vi "NIDAQ-AO-PS_Core.vi"(8 "error in":errorcluster, 10 "ctrl queue in":refnum<queue>) -> (0 "error out":errorcluster, 2 "ctrl queue out":refnum<queue>)   [LabVIEW 2014, in "NIDAQ_AO_PowerSupply.lvlib"]
uses:
  <instrlib>/NIDAQmxAOPowerSupply/NIDAQ_AO_PowerSupply.lvlib
  <instrlib>/GenericDCPowerSupply/Public/GenericDCPS-State.ctl
  <instrlib>/GenericDCPowerSupply/Public/Data/HVCh-Configs.ctl
  <vilib>/Utility/error.llb/Error Cluster From Error Code.vi
  <vilib>/DAQmx/write.llb/DAQmx Write.vi
  <vilib>/DAQmx/write.llb/DAQmx Write (Analog 1D DBL NChan 1Samp).vi
  <vilib>/ErrorRing/Error Ring.xnode
  <userlib>/Utility/ErrorLog_lib.lvlib
  <instrlib>/GenericDCPowerSupply/GenericDCPowerSupply.lvlib
panel:
  out "Power Supply Monitoring":cluster{"Gauge":dbl, "Clamped":bool}[][](array[cluster]) {"Gauge" scale=0.0..5000.0 scale format="%#_6p"}
  in  "Configs":T2={"Enable"=FALSE, "ZeroShutdown"=FALSE, "Initialized"=FALSE, "Configs"=[{"MaxVolt"=5.0, "MinVolt"=0.0, "SetPoint"=0.0, "Readout"=0.0, "Enable"=TRUE, "Channel"=0, "Clamped"=FALSE}, {"MaxVolt"=5.0, "MinVolt"=0.0, "SetPoint"=0.0, "Readout"=0.0, "Enable"=TRUE, "Channel"=1, "Clamped"=FALSE}, {"MaxVolt"=5.0, "MinVolt"=0.0, "SetPoint"=0.0, "Readout"=0.0, "Enable"=TRUE, "Channel"=2, "Clamped"=FALSE}, {"MaxVolt"=5.0, "MinVolt"=0.0, "SetPoint"=0.0, "Readout"=0.0, "Enable"=TRUE, "Channel"=3, "Clamped"=FALSE}, {"MaxVolt"=5.0, "MinVolt"=0.0, "SetPoint"=0.0, "Readout"=0.0, "Enable"=TRUE, "Channel"=4, "Clamped"=FALSE}, {"MaxVolt"=5.0, "MinVolt"=0.0, "SetPoint"=0.0, "Readout"=0.0, "Enable"=TRUE, "Channel"=5, "Clamped"=FALSE}, {"MaxVolt"=5.0, "MinVolt"=0.0, "SetPoint"=0.0, "Readout"=0.0, "Enable"=TRUE, "Channel"=6, "Clamped"=FALSE}, {"MaxVolt"=5.0, "MinVolt"=0.0, "SetPoint"=0.0, "Readout"=0.0, "Enable"=TRUE, "Channel"=7, "Clamped"=FALSE}, {"MaxVolt"=5.0, "MinVolt"=0.0, "SetPoint"=0.0, "Readout"=0.0, "Enable"=TRUE, "Channel"=8, "Clamped"=FALSE}, {"MaxVolt"=5.0, "MinVolt"=0.0, "SetPoint"=0.0, "Readout"=0.0, "Enable"=TRUE, "Channel"=9, "Clamped"=FALSE}, {"MaxVolt"=5.0, "MinVolt"=0.0, "SetPoint"=0.0, "Readout"=0.0, "Enable"=TRUE, "Channel"=10, "Clamped"=FALSE}, {"MaxVolt"=5.0, "MinVolt"=0.0, "SetPoint"=0.0, "Readout"=0.0, "Enable"=TRUE, "Channel"=11, "Clamped"=FALSE}, {"MaxVolt"=5.0, "MinVolt"=0.0, "SetPoint"=0.0, "Readout"=0.0, "Enable"=TRUE, "Channel"=12, "Clamped"=FALSE}, {"MaxVolt"=5.0, "MinVolt"=0.0, "SetPoint"=0.0, "Readout"=0.0, "Enable"=TRUE, "Channel"=13, "Clamped"=FALSE}, {"MaxVolt"=5.0, "MinVolt"=0.0, "SetPoint"=0.0, "Readout"=0.0, "Enable"=TRUE, "Channel"=14, "Clamped"=FALSE}, {"MaxVolt"=5.0, "MinVolt"=0.0, "SetPoint"=0.0, "Readout"=0.0, "Enable"=TRUE, "Channel"=15, "Clamped"=FALSE}], "AO Task Name"="", "# Channels"=16, "Actual Ctrl Voltages"=[]}
  in  "Quit":bool
  in  "SetAll":bool
  # "Copyright (C) 2015 MassThink.\nCopyright (C) 2015 University of Illinois at Chicago\nLicensed under LGPL v3.\n\nProvided AS IS, use at your own risk.\n\nHardware overvoltage protection \nmust be used."
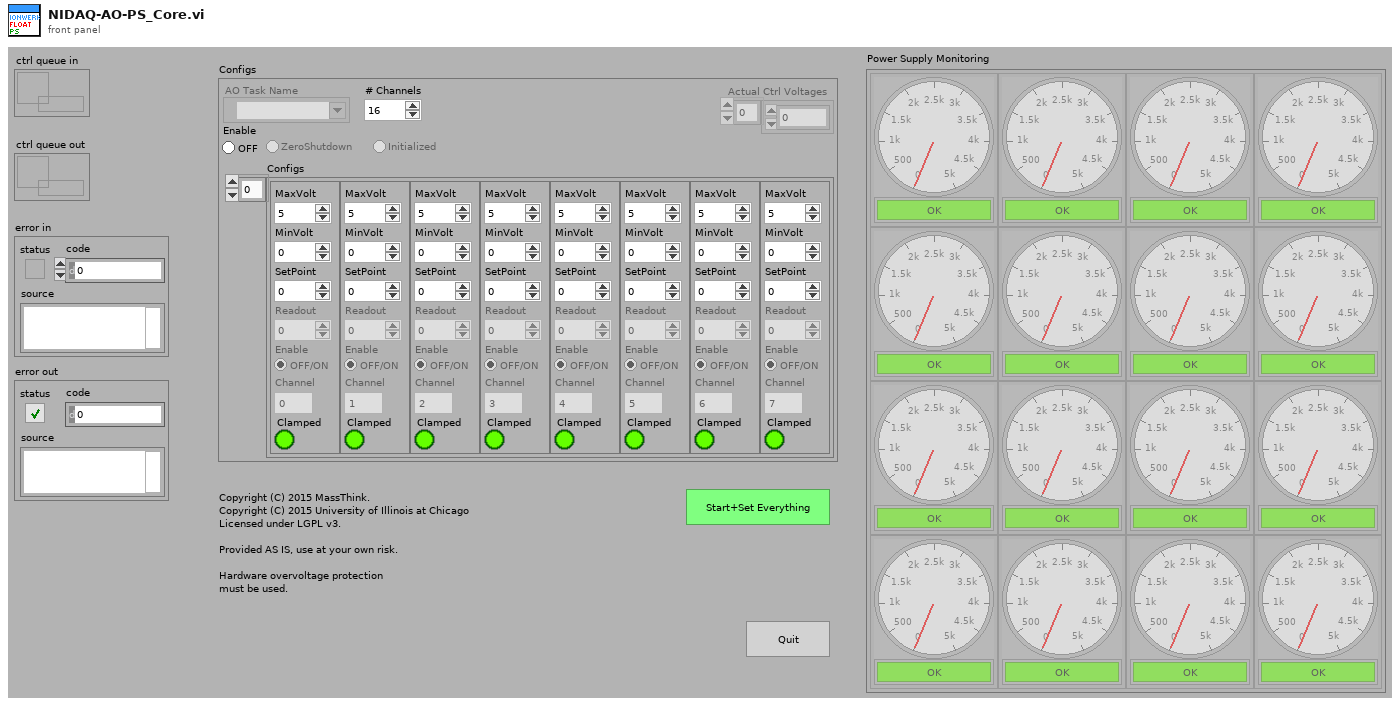
[diagram p1: front panel]
types:
  T1 = typedef "GenericDCPowerSupply.lvlib/HVCh-Configs.ctl" = cluster{"MaxVolt":dbl, "MinVolt":dbl, "SetPoint":dbl, "Readout":dbl, "Enable":bool, "Channel":i32, "Clamped":bool}
  T2 = cluster{"Enable":bool, "ZeroShutdown":bool, "Initialized":bool, "Configs":T1[], "AO Task Name":refnum<k21>, "# Channels":i32, "Actual Ctrl Voltages":dbl[]}
  T3 = enum8{"Enabled", "Disabled", "Disabled and Grayed Out"}
  T4 = cluster{"Slope(Output)":dbl, "Offset(Output)":dbl, "Slope(Input)":dbl, "Offset(Input)":dbl}[][]
  T5 = cluster{"Slope(Output)":dbl, "Offset(Output)":dbl, "Slope(Input)":dbl, "Offset(Input)":dbl}[]
  T6 = typedef "GenericDCPowerSupply.lvlib/GenericDCPS-State.ctl" = cluster{"State":enum16{"Enurmerate", "Open", "WriteVoltage", "ReadVoltage", "WriteAllChs", "ReadAllChs", "OnOff", "SetMinMax", "Close", "Quit", "=========", "GetStatus"}, "Para.":variant}
  T7 = enum16{"Enurmerate", "Open", "WriteVoltage", "ReadVoltage", "WriteAllChs", "ReadAllChs", "OnOff", "SetMinMax", "Close", "Quit", "=========", "GetStatus"}
  T8 = cluster{"Slope(Output)":dbl, "Offset(Output)":dbl, "Slope(Input)":dbl, "Offset(Input)":dbl}
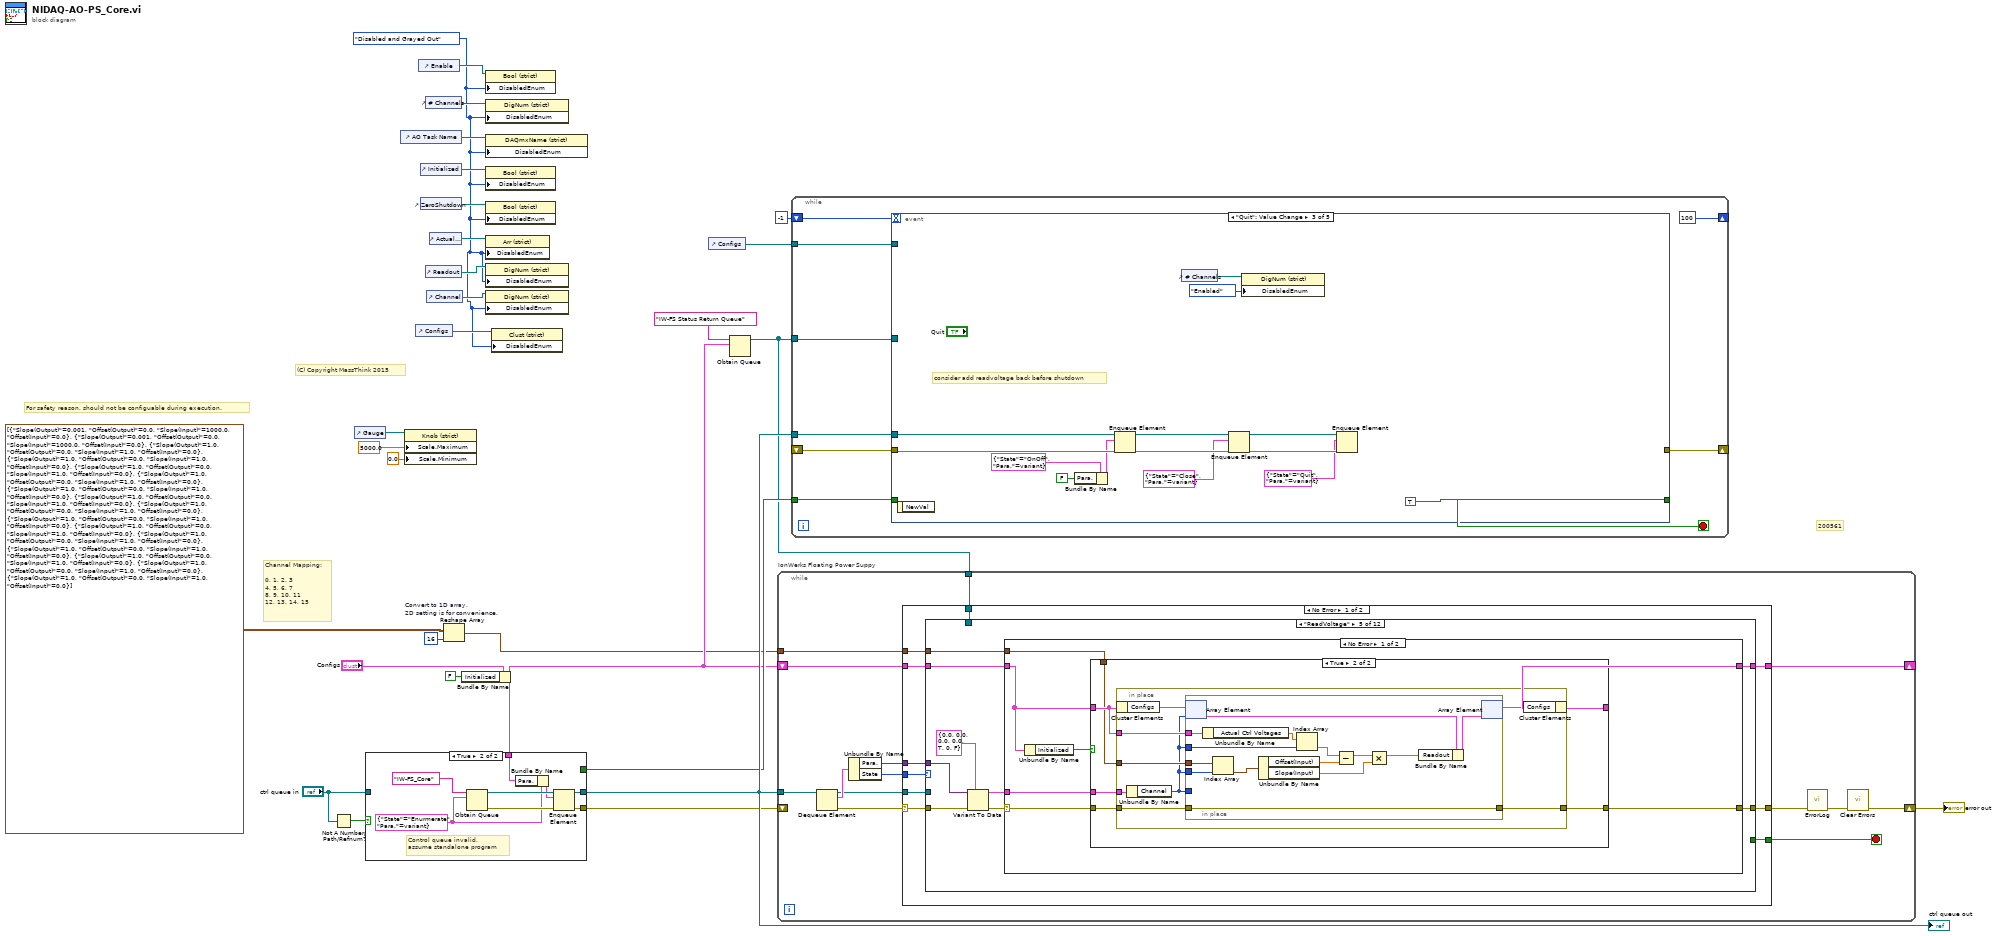
[diagram p0: block diagram]
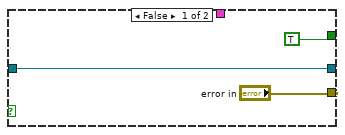
[diagram p2: hidden frame]
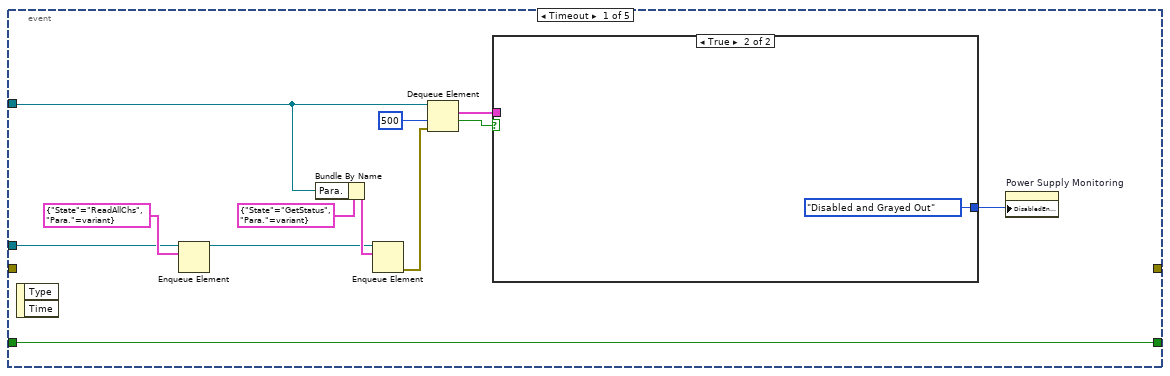
[diagram p3: hidden frame]
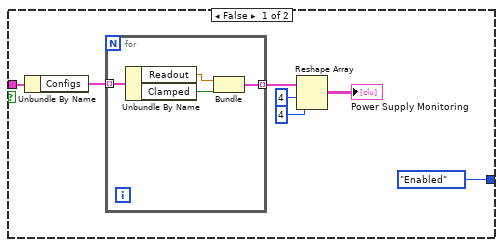
[diagram p4: hidden frame]
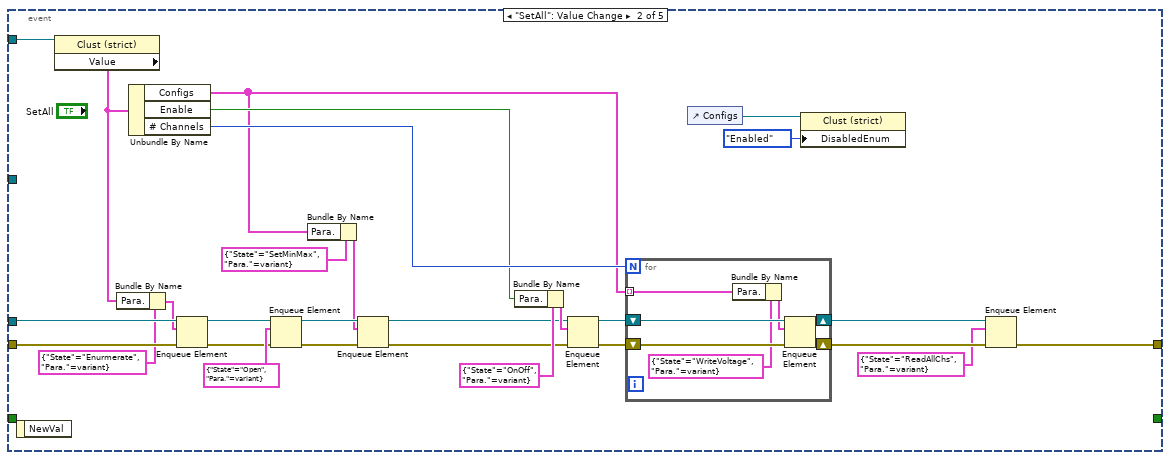
[diagram p5: hidden frame]
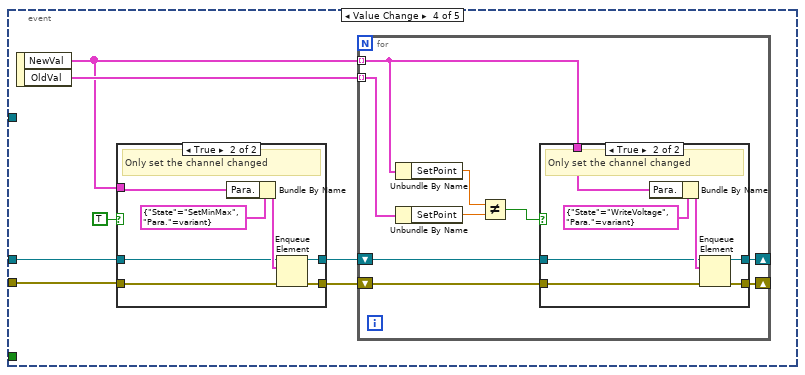
[diagram p6: hidden frame]
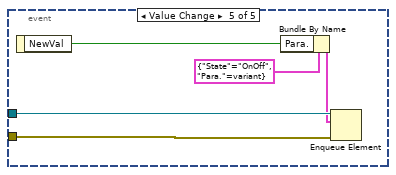
[diagram p9: hidden frame]
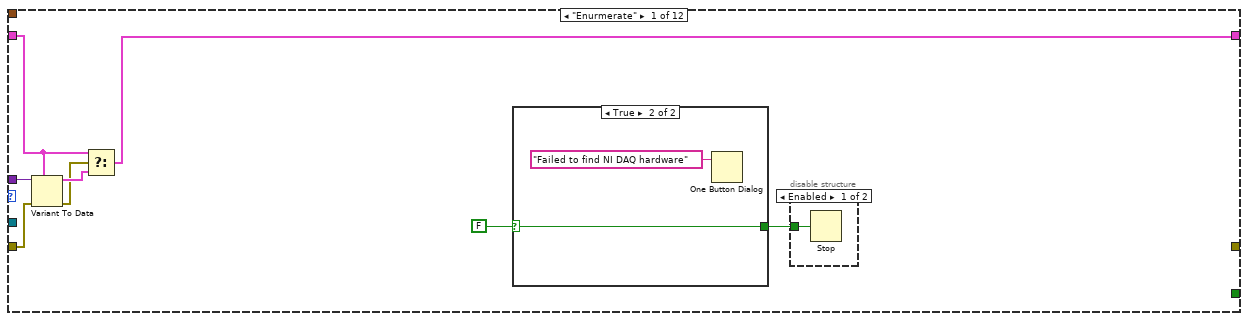
[diagram p10: hidden frame]
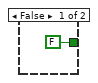
[diagram p12: hidden frame]
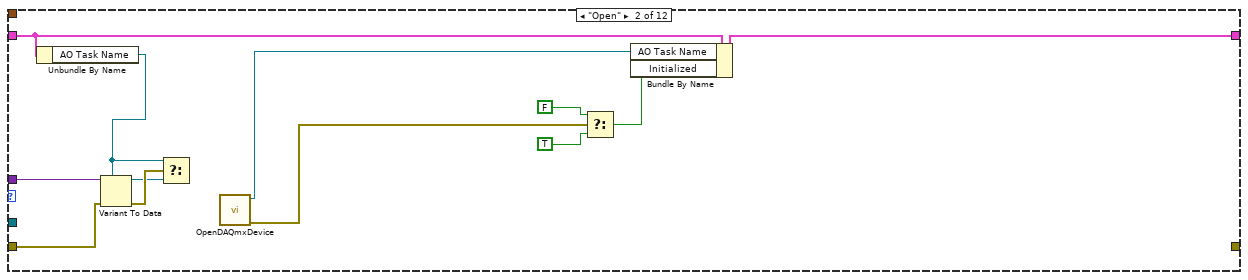
[diagram p13: hidden frame]
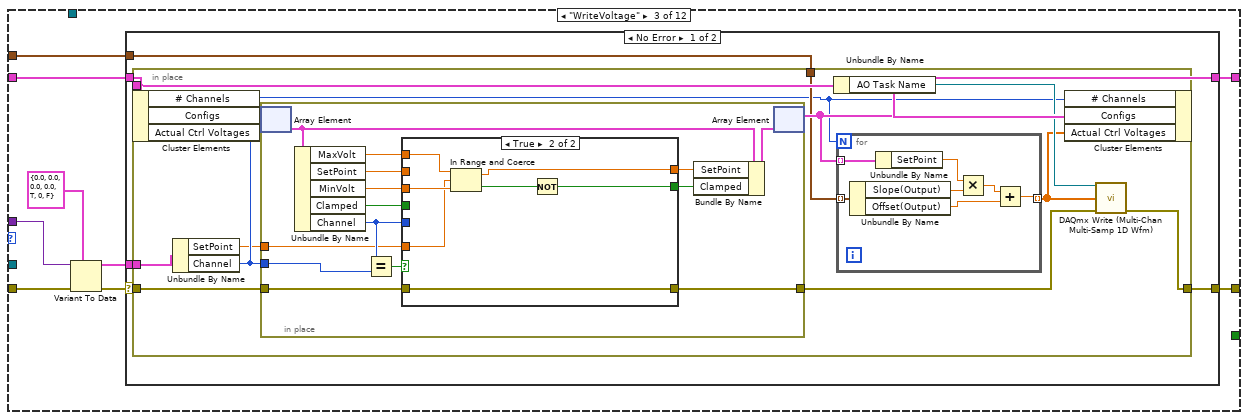
[diagram p14: hidden frame]
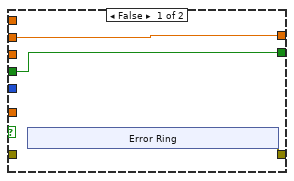
[diagram p15: hidden frame]
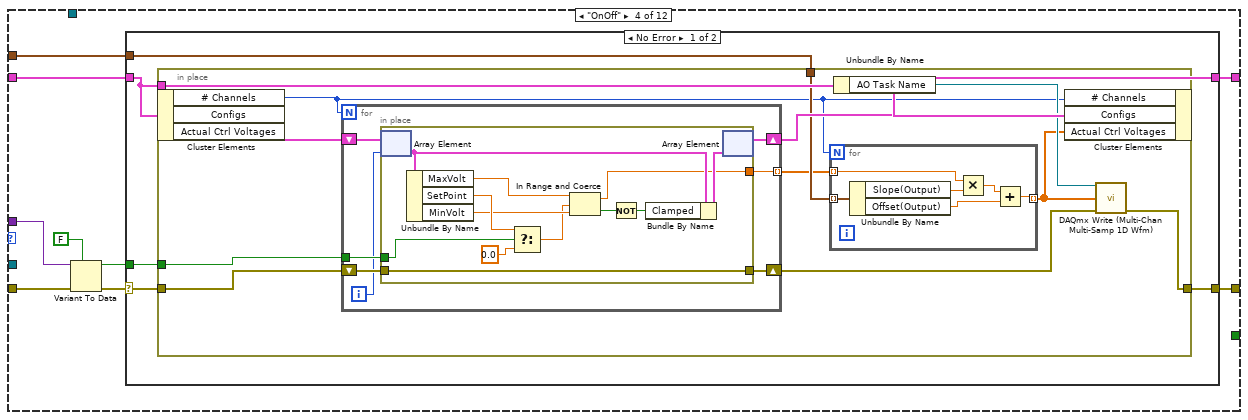
[diagram p17: hidden frame]
diagram:
  w1 = T3."Disabled and Grayed Out" ("Disabled")
  # "200561"
  # "Channel Mapping:\n\n0, 1, 2, 3\n4, 5, 6, 7\n8, 9, 10, 11\n12, 13, 14, 15"
  # "For safety reason, should not be configuable during execution."
  # "(C) Copyright MassThink 2015"
  n1 = Not A Number/Path/Refnum?(number/path/refnum="ctrl queue in") -> (NaN/Path/Refnum?=w28:bool)
  n2 = control-ref of="Gauge"() -> (w20:refnum<vi>)
  n3 = control-ref of="AO Task Name"() -> (w6:refnum<vi>)
  n4 = property class="Knob (strict)"(reference=w20, "Scale.Maximum"=5000.0 ("Scale.Range:Maximum"), "Scale.Minimum"=0.0 ("Scale.Range:Minimum")) -> ()  [unwired: 1 in, 2 out]
  n5 = control-ref of="Configs"() -> (w2:refnum<vi>)
  n6 = control-ref of="Enable"() -> (w5:refnum<vi>)
  n7 = control-ref of="Initialized"() -> (w7:refnum<vi>)
  n8 = control-ref of="ZeroShutdown"() -> (w8:refnum<vi>)
  n9 = control-ref of="# Channels"() -> (w10:refnum<vi>)
  n10 = control-ref of="Readout"() -> (w3:refnum<vi>)
  n11 = control-ref of="Channel"() -> (w4:refnum<vi>)
  n12 = control-ref of="Actual Ctrl Voltages"() -> (w9:refnum<vi>)
  n13 = Reshape Array "Convert to 1D array,\n2D setting is for convenience."(T4 [[{"Slope(Output)"=0.001, "Offset(Output)"=0.0, "Slope(Input)"=1000.0, "Offset(Input)"=0.0}, {"Slope(Output)"=0.001, "Offset(Output)"=0.0, "Slope(Input)"=1000.0, "Offset(Input)"=0.0}, {"Slope(Output)"=1.0, "Offset(Output)"=0.0, "Slope(Input)"=1.0, "Offset(Input)"=0.0}, {"Slope(Output)"=1.0, "Offset(Output)"=0.0, "Slope(Input)"=1.0, "Offset(Input)"=0.0}], [{"Slope(Output)"=1.0, "Offset(Output)"=0.0, "Slope(Input)"=1.0, "Offset(Input)"=0.0}, {"Slope(Output)"=1.0, "Offset(Output)"=0.0, "Slope(Input)"=1.0, "Offset(Input)"=0.0}, {"Slope(Output)"=1.0, "Offset(Output)"=0.0, "Slope(Input)"=1.0, "Offset(Input)"=0.0}, {"Slope(Output)"=1.0, "Offset(Output)"=0.0, "Slope(Input)"=1.0, "Offset(Input)"=0.0}], [{"Slope(Output)"=1.0, "Offset(Output)"=0.0, "Slope(Input)"=1.0, "Offset(Input)"=0.0}, {"Slope(Output)"=1.0, "Offset(Output)"=0.0, "Slope(Input)"=1.0, "Offset(Input)"=0.0}, {"Slope(Output)"=1.0, "Offset(Output)"=0.0, "Slope(Input)"=1.0, "Offset(Input)"=0.0}, {"Slope(Output)"=1.0, "Offset(Output)"=0.0, "Slope(Input)"=1.0, "Offset(Input)"=0.0}], [{"Slope(Output)"=1.0, "Offset(Output)"=0.0, "Slope(Input)"=1.0, "Offset(Input)"=0.0}, {"Slope(Output)"=1.0, "Offset(Output)"=0.0, "Slope(Input)"=1.0, "Offset(Input)"=0.0}, {"Slope(Output)"=1.0, "Offset(Output)"=0.0, "Slope(Input)"=1.0, "Offset(Input)"=0.0}, {"Slope(Output)"=1.0, "Offset(Output)"=0.0, "Slope(Input)"=1.0, "Offset(Input)"=0.0}]] ("output array"), 16 ("dimension size")) -> (w11:T5)
  n14 = Bundle By Name(cluster="Configs", "Initialized"=FALSE) -> (w17:T2)
  n15 = case shown="True" w28 {
    tunnel: [w32 w37] -> w27
    tunnel: ["error in" w39] -> w26
    tunnel: "ctrl queue in" -> [w32 _]
    tunnel: w17 -> [_ w34]
    tunnel: [TRUE _] -> w25
    frame False {
    }
    frame True {
      w33 = T6 {"State"=enum."Enurmerate", "Para."=variant}
      # "Control queue invalid, \nassume standalone program"
      n16 = Obtain Queue(name (unnamed)="IW-FS_Core", element data type=w33) -> (queue out=w38:refnum<queue>, error out=w39:errorcluster)  [unwired: 3 in, 1 out]
      n17 = Bundle By Name(cluster=w33, "Para."=w34) -> (w35:T6)
      n18 = Enqueue Element(queue=w38, element=w35) -> (queue out=w37:refnum<queue>)  [unwired: 2 in, 2 out]
    }
  }
  "ctrl queue out" <- w27
  n19 = property class="Bool (strict)"(reference=w5, "DisabledEnum"=w1) -> ()  [unwired: 1 in, 2 out]
  n20 = property class="DigNum (strict)"(reference=w10, "DisabledEnum"=w1) -> ()  [unwired: 1 in, 2 out]
  n21 = property class="DAQmxName (strict)"(reference=w6, "DisabledEnum"=w1) -> ()  [unwired: 1 in, 2 out]
  n22 = property class="Bool (strict)"(reference=w7, "DisabledEnum"=w1) -> ()  [unwired: 1 in, 2 out]
  n23 = property class="Bool (strict)"(reference=w8, "DisabledEnum"=w1) -> ()  [unwired: 1 in, 2 out]
  n24 = property class="Arr (strict)"(reference=w9, "DisabledEnum"=w1) -> ()  [unwired: 1 in, 2 out]
  n25 = property class="DigNum (strict)"(reference=w3, "DisabledEnum"=w1) -> ()  [unwired: 1 in, 2 out]
  n26 = property class="DigNum (strict)"(reference=w4, "DisabledEnum"=w1) -> ()  [unwired: 1 in, 2 out]
  n27 = property class="Clust (strict)"(reference=w2, "DisabledEnum"=w1) -> ()  [unwired: 1 in, 2 out]
  n28 = control-ref of="Configs"() -> (w15:refnum<vi>)
  n29 = Obtain Queue(name (unnamed)="IW-FS Status Return Queue", element data type=w17) -> (queue out=w18:refnum<queue>)  [unwired: 3 in, 2 out]
  n30 = while "IonWerks Floating Power Suppy" {
    tunnel: w27 -> [w53]
    shift-right: [w44] -> w29
    shift-left: w26 -> [_]
    shift-right: [w45] -> _
    shift-left: w17 -> [w46]
    tunnel: w18 -> [w41]
    tunnel: w11 -> [w40]
    stop <- w47 stop-if-true
    n31 = Dequeue Element(queue=w53) -> (queue out=w49:refnum<queue>, element=w52:T6, error out=w48:errorcluster)  [unwired: 2 in, 1 out]
    n32 = Unbundle By Name(w52) -> ("Para."=w50:variant, "State"=w51:T7)
    n33 = case shown="No Error" w48 {
      selector: w48 -> [w57 w359]
      tunnel: w51 -> [w63 _]
      tunnel: w50 -> [w62 _]
      tunnel: w49 -> [w61 _]
      tunnel: [w60 w359] -> w42
      tunnel: [w56 TRUE] -> w47
      tunnel: w46 -> [w59 w360]
      tunnel: [w58 w360] -> w45
      tunnel: w41 -> [w55 _]
      tunnel: w40 -> [w54 _]
      frame No Error {
        n34 = case shown="\"ReadVoltage\"" w63 {
          tunnel: w62 -> [w71 w87 w95 w162 w215 _ _ w286 _ _ _ w352]
          tunnel: w61 -> [_ _ _ _ _ _ _ _ _ _ _ _]
          tunnel: w57 -> [w70 w85 w94 w161 w214 w258 w263 w285 w329 w348 w350 w354]
          tunnel: [_ _ w89 w156 w210 w258 w262 w283 w328 w348 w350 w353] -> w60
          tunnel: w59 -> [w68 w84 w91 w158 w209 w257 w267 w280 w330 w347 w349 w356]
          tunnel: [w66 w86 w90 w157 w211 w257 w265 w279 w326 w347 w349 w356] -> w58
          tunnel: [_ _ _ _ _ _ _ _ _ TRUE _ _] -> w56
          tunnel: w55 -> [_ _ _ _ _ _ _ _ _ _ _ w351]
          tunnel: w54 -> [_ _ w88 w155 w208 _ w259 _ _ _ _ _]
          frame "Enurmerate" {
            n35 = Variant To Data(error in=w70, type=w68, Variant=w71) -> (data=w69:T2, error out=w67:errorcluster)
            n36 = Select(t=w68, s=w67, f=w69) -> (s? t:f=w66:T2)
            n37 = case shown="True" FALSE ("status") {
              selector: FALSE ("status") -> [_ w74]
              tunnel: [FALSE w74] -> w65
              frame False {
              }
              frame True {
                n38 = One Button Dialog(message="Failed to find NI DAQ hardware") -> ()  [unwired: 1 in, 1 out]
              }
            }
            n39 = disable-structure shown="Enabled" {
              disable-tunnel: w65 -> [w72 _]
              frame Enabled {
                n40 = Stop(stop? (T)=w72) -> ()
              }
              frame Disabled {
              }
            }
          }
          frame "Open" {
            n41 = Unbundle By Name(w84) -> ("AO Task Name"=w82:refnum<k21>)
            n42 = Variant To Data(error in=w85, type=w82, Variant=w87) -> (data=w81:refnum<k21>, error out=w83:errorcluster)
            n43 = Select(t=w82, s=w83, f=w81) -> ()  [unwired: 1 out]
            n44 = call <instrlib>:"OpenDAQmxDevice.vi"() -> ("error out"=w76:errorcluster, "task out"=w77:refnum<k21>)  [unwired: 9 in, 1 out]
            n45 = Select(t=FALSE ("x < y?"), s=w76, f=TRUE ("x < y?")) -> (s? t:f=w80:bool)
            n46 = Bundle By Name(cluster=w84, "AO Task Name"=w77, "Initialized"=w80) -> (w86:T2)
          }
          frame "WriteVoltage" {
            n47 = Variant To Data(error in=w94, type=T1 {"MaxVolt"=0.0, "MinVolt"=0.0, "SetPoint"=0.0, "Readout"=0.0, "Enable"=TRUE, "Channel"=0, "Clamped"=FALSE}, Variant=w95) -> (data=w92:T1, error out=w93:errorcluster)
            n48 = case shown="No Error" w93 {
              selector: w93 -> [w99 w153]
              tunnel: w92 -> [w101 _]
              tunnel: w91 -> [w98 w152]
              tunnel: [w102 w152] -> w90
              tunnel: [w100 w153] -> w89
              tunnel: w88 -> [w97 _]
              frame No Error {
                n49 = in-place {
                  in-place-border: w101 -> [w114]
                  in-place-border: [w106] -> w100
                  in-place-border: w99 -> [w112]
                  in-place-border: w98 -> [w108]
                  in-place-border: w97 -> [w105]
                  n50 = in-place-cluster #1(w98) -> ("# Channels"=w104:i32, "Configs"=w115:T1[])  [unwired: 1 out]
                  n51 = Unbundle By Name(w114) -> ("SetPoint"=w111:dbl, "Channel"=w113:i32)
                  n52 = in-place {
                    in-place-border: w113 -> [w136]
                    in-place-border: [w128] -> w107
                    in-place-border: w112 -> [w127]
                    in-place-border: w111 -> [w123]
                    n53 = in-place-array #2(w115, w113) -> (w130:T1)
                    n54 = Unbundle By Name(w130) -> ("MaxVolt"=w132:dbl, "SetPoint"=w134:dbl, "MinVolt"=w133:dbl, "Clamped"=w125:bool, "Channel"=w124:i32)
                    n55 = Equal?(x=w124, y=w136) -> (x = y?=w135:bool)
                    n56 = case shown="True" w135 {
                      tunnel: w134 -> [w139 _]
                      tunnel: w133 -> [_ w151]
                      tunnel: w132 -> [_ w150]
                      tunnel: [w139 w148] -> w129
                      tunnel: [w138 w147] -> w128
                      tunnel: w127 -> [_ w147]
                      tunnel: [w137 w146] -> w126
                      tunnel: w125 -> [w137 _]
                      tunnel: w124 -> [_ _]
                      tunnel: w123 -> [_ w145]
                      frame False {
                        n57 = xnode "Error Ring"() -> ("error out"=w138:errorcluster)
                      }
                      frame True {
                        n58 = In Range and Coerce(upper limit=w150, x=w145, lower limit=w151) -> (coerced(x)=w148:dbl, In Range?=w149:bool)
                        n59 = Not(x=w149) -> (.not. x?=w146:bool)
                      }
                    }
                    n60 = Bundle By Name(cluster=w130, "SetPoint"=w129, "Clamped"=w126) -> (w131:T1)
                    n61 = in-place-array #2(w131) -> (w110:T1[])  [unwired: 1 out]
                  }
                  n62 = Unbundle By Name(w108) -> ("AO Task Name"=w109:refnum<k21>)
                  n63 = for {
                    N: w104 -> [_]
                    tunnel: w110 -> [w122] mode=indexing
                    tunnel: [w116] -> w103 mode=indexing
                    tunnel: w105 -> [w121] mode=indexing
                    n64 = Unbundle By Name(w121) -> ("Slope(Output)"=w120:dbl, "Offset(Output)"=w118:dbl)
                    n65 = Unbundle By Name(w122) -> ("SetPoint"=w119:dbl)
                    n66 = Multiply(x=w119, y=w120) -> (x*y=w117:dbl)
                    n67 = Add(x=w117, y=w118) -> (x+y=w116:dbl)
                  }
                  n68 = in-place-cluster #1("# Channels"=w104, "Configs"=w110, "Actual Ctrl Voltages"=w103) -> (w102:T2)
                  n69 = call-poly "DAQmx Write (Multi-Chan Multi-Samp 1D Wfm).vi"("task/channels in"=w109, "data"=w103, "error in"=w107) -> ("error out"=w106:errorcluster)  [unwired: 10 in, 2 out]
                }
              }
              frame Error {
              }
            }
          }
          frame "OnOff" {
            n70 = Variant To Data(error in=w161, type=FALSE, Variant=w162) -> (data=w159:bool, error out=w160:errorcluster)
            n71 = case shown="No Error" w160 {
              selector: w160 -> [w165 w207]
              tunnel: w159 -> [w167 _]
              tunnel: w158 -> [w164 w206]
              tunnel: [w168 w206] -> w157
              tunnel: [w166 w207] -> w156
              tunnel: w155 -> [w163 _]
              frame No Error {
                n72 = in-place {
                  in-place-border: w167 -> [w173]
                  in-place-border: [w175] -> w166
                  in-place-border: w165 -> [w180]
                  in-place-border: w164 -> [w177]
                  in-place-border: w163 -> [w174]
                  n73 = in-place-cluster #3(w164) -> ("# Channels"=w171:i32, "Configs"=w172:T1[])  [unwired: 1 out]
                  n74 = for {
                    N: w171 -> [_]
                    tunnel: w173 -> [w183]
                    shift-right: [w184] -> w176
                    shift-left: w180 -> [w186]
                    shift-right: [w185] -> w179
                    shift-left: w172 -> [w187]
                    tunnel: [w181] -> w170 mode=indexing
                    i -> [w182]
                    n75 = in-place {
                      in-place-border: [w194] -> w184
                      in-place-border: w186 -> [w194]
                      in-place-border: w183 -> [w192]
                      in-place-border: [w188] -> w181
                      n76 = in-place-array #4(w187, w182) -> (w195:T1)
                      n77 = Unbundle By Name(w195) -> ("MaxVolt"=w197:dbl, "SetPoint"=w199:dbl, "MinVolt"=w198:dbl)
                      n78 = Select(t=w199, s=w192, f=0.0 ("x")) -> (s? t:f=w190:dbl)
                      n79 = In Range and Coerce(upper limit=w197, x=w190, lower limit=w198) -> (coerced(x)=w188:dbl, In Range?=w191:bool)
                      n80 = Not(x=w191) -> (.not. x?=w193:bool)
                      n81 = Bundle By Name(cluster=w195, "Clamped"=w193) -> (w196:T1)
                      n82 = in-place-array #4(w196) -> (w185:T1[])  [unwired: 1 out]
                    }
                  }
                  n83 = for {
                    N: w171 -> [_]
                    tunnel: [w201] -> w169 mode=indexing
                    tunnel: w174 -> [w205] mode=indexing
                    tunnel: w170 -> [w200] mode=indexing
                    n84 = Unbundle By Name(w205) -> ("Slope(Output)"=w204:dbl, "Offset(Output)"=w203:dbl)
                    n85 = Multiply(x=w200, y=w204) -> (x*y=w202:dbl)
                    n86 = Add(x=w202, y=w203) -> (x+y=w201:dbl)
                  }
                  n87 = Unbundle By Name(w177) -> ("AO Task Name"=w178:refnum<k21>)
                  n88 = in-place-cluster #3("# Channels"=w171, "Configs"=w179, "Actual Ctrl Voltages"=w169) -> (w168:T2)
                  n89 = call-poly "DAQmx Write (Multi-Chan Multi-Samp 1D Wfm).vi"("task/channels in"=w178, "data"=w169, "error in"=w176) -> ("error out"=w175:errorcluster)  [unwired: 10 in, 2 out]
                }
              }
              frame Error {
              }
            }
          }
          frame "ReadVoltage" {
            n90 = Variant To Data(error in=w214, type=T1 {"MaxVolt"=0.0, "MinVolt"=0.0, "SetPoint"=0.0, "Readout"=0.0, "Enable"=TRUE, "Channel"=0, "Clamped"=FALSE}, Variant=w215) -> (data=w212:T1, error out=w213:errorcluster)
            n91 = case shown="No Error" w213 {
              selector: w213 -> [w220 w255]
              tunnel: w212 -> [w222 _]
              tunnel: w209 -> [w219 w254]
              tunnel: [w223 w254] -> w211
              tunnel: [w221 w255] -> w210
              tunnel: w208 -> [w217 _]
              frame No Error {
                n92 = Unbundle By Name(w219) -> ("Initialized"=w218:bool)
                n93 = case shown="True" w218 {
                  tunnel: [w225 w231] -> w223
                  tunnel: w222 -> [_ w230]
                  tunnel: [w224 w229] -> w221
                  tunnel: w220 -> [w224 w228]
                  tunnel: w219 -> [w225 w227]
                  tunnel: w217 -> [_ w226]
                  frame False {
                  }
                  frame True {
                    n94 = in-place {
                      in-place-border: w230 -> [w237]
                      in-place-border: [w236] -> w229
                      in-place-border: w228 -> [w235]
                      in-place-border: w227 -> [w234]
                      in-place-border: w226 -> [w233]
                      n95 = in-place-cluster #5(w227) -> ("Configs"=w239:T1[])
                      n96 = Unbundle By Name(w237) -> ("Channel"=w232:i32)
                      n97 = in-place {
                        in-place-border: w232 -> [_]
                        in-place-border: [w252] -> w236
                        in-place-border: w235 -> [w252]
                        in-place-border: w234 -> [w250]
                        in-place-border: w232 -> [w248]
                        in-place-border: w233 -> [w244]
                        in-place-border: w232 -> [w243]
                        n98 = in-place-array #6(w239, w232) -> (w251:T1)
                        n99 = Unbundle By Name(w250) -> ("Actual Ctrl Voltages"=w249:dbl[])
                        n100 = Index Array(array=w244, index=w243) -> (element=w242:T8)
                        n101 = Unbundle By Name(w242) -> ("Offset(Input)"=w241:dbl, "Slope(Input)"=w240:dbl)
                        n102 = Index Array(array=w249, index=w248) -> (element=w247:dbl)
                        n103 = Subtract(x=w247, y=w241) -> (x-y=w246:dbl)
                        n104 = Multiply(x=w246, y=w240) -> (x*y=w245:dbl)
                        n105 = Bundle By Name(cluster=w251, "Readout"=w245) -> (w253:T1)
                        n106 = in-place-array #6(w253) -> (w238:T1[])  [unwired: 1 out]
                      }
                      n107 = in-place-cluster #5("Configs"=w238) -> (w231:T2)
                    }
                  }
                }
              }
              frame Error {
              }
            }
          }
          frame "WriteAllChs" {
            n108 = One Button Dialog(message="Write all channel is not implemented yet. ") -> ()  [unwired: 1 in, 1 out]
          }
          frame "ReadAllChs" {
            n109 = Unbundle By Name(w267) -> ("# Channels"=w261:i32, "Configs"=w266:T1[], "Actual Ctrl Voltages"=w260:dbl[])
            n110 = for {
              N: w261 -> [_]
              tunnel: w263 -> [w276]
              tunnel: [w276] -> w262
              tunnel: w266 -> [w274] mode=indexing
              tunnel: [w275] -> w264 mode=indexing
              tunnel: w260 -> [w270] mode=indexing
              tunnel: w259 -> [w269] mode=indexing
              n111 = Unbundle By Name(w269) -> ("Offset(Input)"=w272:dbl, "Slope(Input)"=w271:dbl)
              n112 = Subtract(x=w270, y=w272) -> (x-y=w273:dbl)
              n113 = Multiply(x=w273, y=w271) -> (x*y=w268:dbl)
              n114 = Bundle By Name(cluster=w274, "Readout"=w268) -> (w275:T1)
            }
            n115 = Bundle By Name(cluster=w267, "Configs"=w264) -> (w265:T2)
          }
          frame "SetMinMax" {
            n116 = Unbundle By Name(w280) -> ("# Channels"=w281:i32, "Configs"=w277:T1[])
            n117 = Variant To Data(error in=w285, type=w277, Variant=w286) -> (data=w282:T1[], error out=w284:errorcluster)
            n118 = case shown="No Error" w284 {
              selector: w284 -> [w288 w321]
              tunnel: [w289 w321] -> w283
              tunnel: w282 -> [w292 _]
              tunnel: w281 -> [w291 _]
              tunnel: w277 -> [w290 w320]
              tunnel: [w287 w320] -> w278
              frame No Error {
                n119 = for {
                  N: w291 -> [_]
                  tunnel: w292 -> [w304] mode=indexing
                  tunnel: w290 -> [w298] mode=indexing
                  shift-right: [w300] -> w289
                  shift-left: w288 -> [w299]
                  tunnel: [w297] -> w287 mode=indexing
                  i -> [w302]
                  n120 = Unbundle By Name(w304) -> ("MaxVolt"=w295:dbl, "MinVolt"=w294:dbl, "Channel"=w303:i32)
                  n121 = Unbundle By Name(w298) -> ("MaxVolt"=w296:dbl, "MinVolt"=w293:dbl)
                  n122 = Equal?(x=w303, y=w302) -> (x = y?=w301:bool)
                  n123 = case shown="True" w301 {
                    tunnel: [w309 w319] -> w300
                    tunnel: w299 -> [_ w319]
                    tunnel: w298 -> [w307 w318]
                    tunnel: [w308 w317] -> w297
                    tunnel: w296 -> [w306 _]
                    tunnel: w295 -> [_ w316]
                    tunnel: w294 -> [_ w315]
                    tunnel: w293 -> [w305 _]
                    frame False {
                      n124 = xnode "Error Ring"() -> ("error out"=w309:errorcluster)
                      n125 = Bundle By Name(cluster=w307, "MaxVolt"=w306, "MinVolt"=w305) -> (w308:T1)
                    }
                    frame True {
                      n126 = Bundle By Name(cluster=w318, "MaxVolt"=w316, "MinVolt"=w315) -> (w317:T1)
                    }
                  }
                }
              }
              frame Error {
              }
            }
            n127 = Bundle By Name(cluster=w280, "Configs"=w278) -> (w279:T2)
          }
          frame "Close" {
            n128 = Unbundle By Name(w330) -> ("AO Task Name"=w327:refnum<k21>, "Configs"=w325:T1[], "ZeroShutdown"=w323:bool, "Initialized"=w322:bool)
            n129 = case shown="True" w322 {
              tunnel: w329 -> [w331 w341]
              tunnel: [w331 w335] -> w328
              tunnel: w327 -> [_ w333]
              tunnel: w325 -> [w332 w340]
              tunnel: [w332 w339] -> w324
              tunnel: w323 -> [_ w338]
              frame False {
              }
              frame True {
                n130 = case shown="True" w338 {
                  tunnel: w341 -> [w342 w344]
                  tunnel: [w342 w344] -> w337
                  tunnel: w333 -> [_ _]
                  tunnel: w340 -> [w343 w345]
                  tunnel: [w343 w345] -> w339
                  frame False {
                  }
                  frame True {
                    # "Safety Feature: Shutdown all channel when closes."
                  }
                }
                n131 = call <vilib>:"DAQmx Stop Task.vi"("task/channels in"=w333, "error in"=w337) -> ("task out"=w334:refnum<k21>, "error out"=w336:errorcluster)  [unwired: 12 in]
                n132 = call <vilib>:"DAQmx Clear Task.vi"("task in"=w334, "error in"=w336) -> ("error out"=w335:errorcluster)  [unwired: 13 in]
              }
            }
            n133 = Bundle By Name(cluster=w330, "Configs"=w324) -> (w326:T2)
          }
          frame "Quit" {
          }
          frame "=========" {
          }
          frame "GetStatus" {
            n134 = Variant To Data(error in=w354, type=w351, Variant=w352) -> (data=w357:refnum<queue>, error out=w355:errorcluster)
            n135 = Enqueue Element(queue=w357, element=w356, error in (no error)=w355) -> (error out=w353:errorcluster)  [unwired: 1 in, 2 out]
          }
        }
      }
      frame Error {
      }
    }
    n136 = call <userlib>:"ErrorLog.vi"("error in (no error)"=w42) -> ("error out"=w43:errorcluster)  [unwired: 10 in]
    n137 = call <vilib>:"Clear Errors.vi"("error in (no error)"=w43) -> ("error out"=w44:errorcluster)  [unwired: 5 in, 1 out]
  }
  "error out" <- w29
  n138 = while {
    tunnel: w27 -> [w369]
    shift-right: [w368] -> _
    shift-left: _ -> [w367]
    tunnel: w25 -> [w365]
    shift-right: [100] -> _
    shift-left: -1 -> [w364]
    tunnel: w18 -> [w362]
    tunnel: w15 -> [w361]
    stop <- w366 stop-if-true
    n139 = event shown="[2] \"Quit\": Value Change" {
      selector: _ -> [_ _ _ _ _]
      dyn-events: _ -> [_ _ _ _ _]
      timeout: w364 -> [_ _ _ _ _]
      tunnel: w369 -> [w371 w421 w440 w449 w481]
      tunnel: [_ w417 _ _ _] -> w368
      tunnel: w367 -> [_ w420 w441 w444 w480]
      tunnel: [w381 _ TRUE _ _] -> w366
      tunnel: w365 -> [w381 _ _ _ _]
      tunnel: w362 -> [w378 _ _ _ _]
      tunnel: w361 -> [_ w416 _ _ _]
      event Timeout {
        n140 = event-data() -> ()  [unwired: 1 in, 2 out]
        n141 = Enqueue Element(queue=w371, element=T6 {"State"=enum."ReadAllChs", "Para."=variant}) -> (queue out=w372:refnum<queue>)  [unwired: 2 in, 2 out]
        n142 = Bundle By Name(cluster=T6 {"State"=enum."GetStatus", "Para."=variant} ("element"), "Para."=w378) -> (w379:T6)
        n143 = Enqueue Element(queue=w372, element=w379) -> (error out=w377:errorcluster)  [unwired: 2 in, 2 out]
        n144 = Dequeue Element(queue=w378, timeout in ms (-1)=500, error in (no error)=w377) -> (element=w376:T2, timed out?=w374:bool)  [unwired: 2 out]
        n145 = case shown="True" w374 {
          tunnel: w376 -> [w388 _]
          tunnel: [T3."Enabled" ("Disabled") T3."Disabled and Grayed Out" ("Disabled")] -> w370
          frame False {
            n146 = Unbundle By Name(w388) -> ("Configs"=w387:T1[])
            n147 = for {
              tunnel: w387 -> [w392] mode=indexing
              tunnel: [w389] -> w386 mode=indexing
              n148 = Unbundle By Name(w392) -> ("Readout"=w391:dbl, "Clamped"=w390:bool)
              n149 = Bundle("Readout"=w391, "Clamped"=w390) -> (w389:cluster{"Readout":dbl, "Clamped":bool})  [unwired: 1 in]
            }
            n150 = Reshape Array(w386, 4 ("dimension size"), 4 ("dimension size")) -> (→"Power Supply Monitoring":cluster{"Readout":dbl, "Clamped":bool}[][])
          }
          frame True {
          }
        }
        n151 = property on="Power Supply Monitoring" class="Arr (strict)"("DisabledEnum"=w370) -> ()  [unwired: 2 in, 2 out]
      }
      event "SetAll": Value Change {
        n152 = event-data() -> ()  [unwired: 1 in, 1 out]
        n153 = property class="Clust (strict)"(reference=w416) -> ("Value"=w406:T2)  [unwired: 1 in, 2 out]
        n154 = Bundle By Name(cluster=T6 {"State"=enum."Enurmerate", "Para."=variant} ("element"), "Para."=w406) -> (w407:T6)
        n155 = Unbundle By Name(w406) -> ("Configs"=w396:T1[], "Enable"=w408:bool, "# Channels"=w415:i32)
        n156 = Enqueue Element(queue=w421, element=w407, error in (no error)=w420) -> (queue out=w412:refnum<queue>, error out=w411:errorcluster)  [unwired: 1 in, 1 out]
        n157 = Enqueue Element(queue=w412, element=T6 {"State"=enum."Open", "Para."=variant}, error in (no error)=w411) -> (queue out=w402:refnum<queue>, error out=w399:errorcluster)  [unwired: 1 in, 1 out]
        n158 = Bundle By Name(cluster=T6 {"State"=enum."SetMinMax", "Para."=variant} ("element"), "Para."=w396) -> (w401:T6)
        n159 = Enqueue Element(queue=w402, element=w401, error in (no error)=w399) -> (queue out=w397:refnum<queue>, error out=w398:errorcluster)  [unwired: 1 in, 1 out]
        n160 = Bundle By Name(cluster=T6 {"State"=enum."OnOff", "Para."=variant} ("element"), "Para."=w408) -> (w409:T6)
        n161 = Enqueue Element(queue=w397, element=w409, error in (no error)=w398) -> (queue out=w404:refnum<queue>, error out=w405:errorcluster)  [unwired: 1 in, 1 out]
        n162 = for {
          N: w415 -> [_]
          shift-right: [w426] -> w418
          shift-left: w405 -> [w427]
          shift-right: [w425] -> w419
          shift-left: w404 -> [w428]
          tunnel: w396 -> [w422] mode=indexing
          n163 = Bundle By Name(cluster=T6 {"State"=enum."WriteVoltage", "Para."=variant} ("element"), "Para."=w422) -> (w424:T6)
          n164 = Enqueue Element(queue=w428, element=w424, error in (no error)=w427) -> (queue out=w425:refnum<queue>, error out=w426:errorcluster)  [unwired: 1 in, 1 out]
        }
        n165 = control-ref of="Configs"() -> (w395:refnum<vi>)
        n166 = property class="Clust (strict)"(reference=w395, "DisabledEnum"=T3."Enabled" ("Disabled")) -> ()  [unwired: 1 in, 2 out]
        n167 = Enqueue Element(queue=w419, element=T6 {"State"=enum."ReadAllChs", "Para."=variant}, error in (no error)=w418) -> (error out=w417:errorcluster)  [unwired: 1 in, 2 out]
      }
      event "Quit": Value Change {
        # "consider add readvoltage back before shutdown"
        n168 = event-data() -> ()  [unwired: 1 in, 1 out]
        n169 = Bundle By Name(cluster=T6 {"State"=enum."OnOff", "Para."=variant}, "Para."=FALSE) -> (w434:T6)
        n170 = Enqueue Element(queue=w440, element=w434, error in (no error)=w441) -> (queue out=w437:refnum<queue>, error out=w436:errorcluster)  [unwired: 1 in, 1 out]
        n171 = control-ref of="# Channels"() -> (w430:refnum<vi>)
        n172 = Enqueue Element(queue=w437, element=T6 {"State"=enum."Close", "Para."=variant}, error in (no error)=w436) -> (queue out=w439:refnum<queue>, error out=w438:errorcluster)  [unwired: 1 in, 1 out]
        n173 = property class="DigNum (strict)"(reference=w430, "DisabledEnum"=T3."Enabled" ("Disabled")) -> ()  [unwired: 1 in, 2 out]
        n174 = Enqueue Element(queue=w439, element=T6 {"State"=enum."Quit", "Para."=variant}, error in (no error)=w438) -> ()  [unwired: 1 in, 3 out]
      }
      event "Configs.Configs": Value Change {
        n175 = event-data() -> ("NewVal"=w446:T1[], "OldVal"=w447:T1[])  [unwired: 1 in]
        n176 = case shown="True" TRUE {
          tunnel: w446 -> [_ w456]
          tunnel: w449 -> [w451 w455]
          tunnel: [w451 w454] -> w443
          tunnel: w444 -> [w450 w453]
          tunnel: [w450 w452] -> w448
          frame False {
          }
          frame True {
            # "Only set the channel changed"
            n177 = Bundle By Name(cluster=T6 {"State"=enum."SetMinMax", "Para."=variant} ("element"), "Para."=w456) -> (w458:T6)
            n178 = Enqueue Element(queue=w455, element=w458, error in (no error)=w453) -> (queue out=w454:refnum<queue>, error out=w452:errorcluster)  [unwired: 1 in, 1 out]
          }
        }
        n179 = for {
          tunnel: w446 -> [w464] mode=indexing
          tunnel: w447 -> [w467] mode=indexing
          shift-right: [w460] -> _
          shift-left: w448 -> [w461]
          shift-right: [w459] -> _
          shift-left: w443 -> [w462]
          n180 = Unbundle By Name(w464) -> ("SetPoint"=w466:dbl)
          n181 = Unbundle By Name(w467) -> ("SetPoint"=w465:dbl)
          n182 = Not Equal?(x=w466, y=w465) -> (x != y?=w463:bool)
          n183 = case shown="True" w463 {
            tunnel: w464 -> [_ w474]
            tunnel: w462 -> [w468 w473]
            tunnel: w461 -> [w469 w472]
            tunnel: [w469 w471] -> w460
            tunnel: [w468 w470] -> w459
            frame False {
            }
            frame True {
              # "Only set the channel changed"
              n184 = Bundle By Name(cluster=T6 {"State"=enum."WriteVoltage", "Para."=variant} ("element"), "Para."=w474) -> (w476:T6)
              n185 = Enqueue Element(queue=w473, element=w476, error in (no error)=w472) -> (queue out=w470:refnum<queue>, error out=w471:errorcluster)  [unwired: 1 in, 1 out]
            }
          }
        }
      }
      event "Configs.Enable": Value Change {
        n186 = event-data() -> ("NewVal"=w479:bool)  [unwired: 1 in]
        n187 = Bundle By Name(cluster=T6 {"State"=enum."OnOff", "Para."=variant} ("element"), "Para."=w479) -> (w478:T6)
        n188 = Enqueue Element(queue=w481, element=w478, error in (no error)=w480) -> ()  [unwired: 1 in, 3 out]
      }
    }
  }
